vi "Write Status Calculation.vi"(8 "error in (no error)":errorcluster, 10 "Status Calculation":T1, 11 "abs_Parallel in":refnum<class "abs_Parallel.lvclass">) -> (0 "error out":errorcluster, 3 "abs_Parallel out":refnum<class "abs_Parallel.lvclass">)   [LabVIEW 2021, in "BT.lvlib" / "abs_Parallel.lvclass"]
uses:
  abs_Parallel.lvclass
  abs_Parallel.lvclass/abs_Parallel.ctl
  Support/Status Calculation.ctl
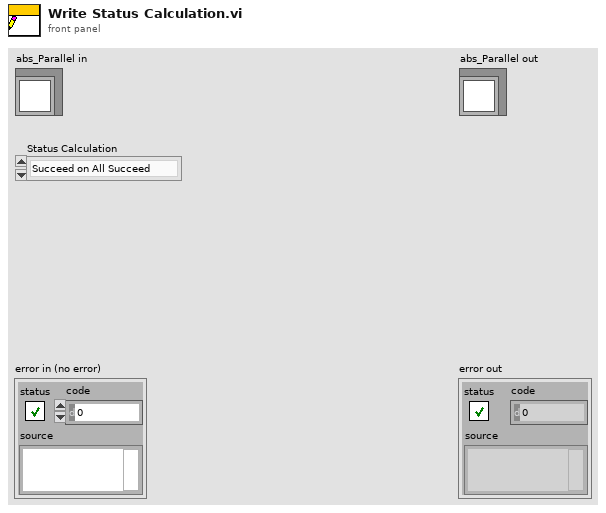
[diagram p1: front panel]
types:
  T1 = typedef "BT.lvlib/abs_Parallel.lvclass/Status Calculation.ctl" = enum16{"Succeed on All Succeed", "Failure on All Failure", "Succeed on Any Succeed", "Failure on Any Failure"}
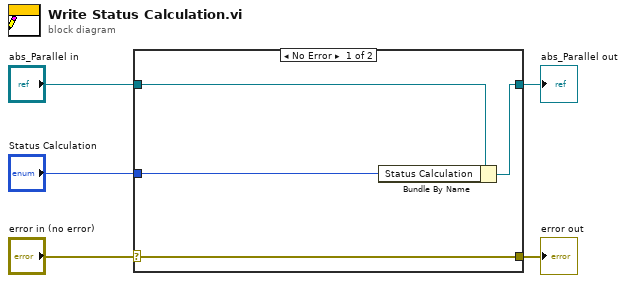
[diagram p0: block diagram]
diagram:
  n1 = case shown="No Error" "error in (no error)" {
    selector: "error in (no error)" -> [w9 w10]
    tunnel: [w9 w10] -> w4
    tunnel: [w7 w11] -> w2
    tunnel: "abs_Parallel in" -> [w8 w11]
    tunnel: "Status Calculation" -> [w6 _]
    frame No Error {
      n2 = Bundle By Name(cluster=w8, "Status Calculation"=w6) -> (w7:refnum<class "abs_Parallel.lvclass">)
    }
    frame Error {
    }
  }
  "error out" <- w4
  "abs_Parallel out" <- w2
